vi "Append String to Error Source.vi"(4 "Append to Warning? (F)":bool, 6 "Prepend? (F)":bool, 8 "Error In":errorcluster, 9 "String to Append":string) -> (0 "Error Out":errorcluster)   [LabVIEW 2023]
doc: "Append or Prepend the specified message to the input error source string if error exists."
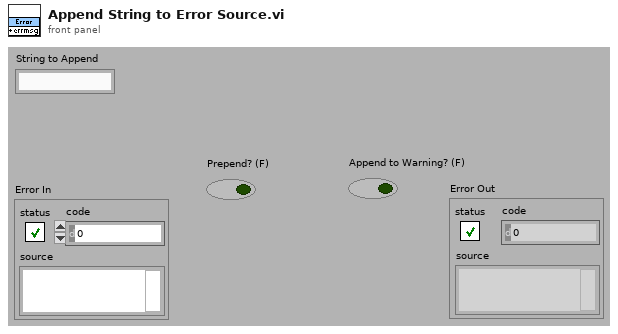
[diagram p1: front panel]
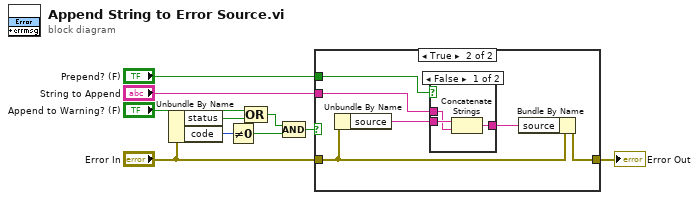
[diagram p0: block diagram]
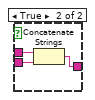
[diagram p3: hidden frame]
diagram:
  n1 = Unbundle By Name("Error In") -> ("status"=w10:bool, "code"=w7:i32)
  n2 = Not Equal To 0?(x=w7) -> (x != 0?=w6:bool)
  n3 = Compound Arithmetic op=OR("Append to Warning? (F)", w10) -> (w8:bool)
  n4 = Compound Arithmetic op=AND(w8, w6) -> (w5:bool)
  n5 = case shown="True" w5 {
    tunnel: "Error In" -> [w11 w17]
    tunnel: [w11 w16] -> w3
    tunnel: "Prepend? (F)" -> [_ w12]
    tunnel: "String to Append" -> [_ w13]
    frame False {
    }
    frame True {
      n6 = Unbundle By Name(w17) -> ("source"=w15:string)
      n7 = case shown="False" w12 {
        tunnel: w15 -> [w20 w23]
        tunnel: [w19 w21] -> w14
        tunnel: w13 -> [w18 w22]
        frame False {
          n8 = Concatenate Strings(w20, w18) -> (w19:string)
        }
        frame True {
          n9 = Concatenate Strings(w22, w23) -> (w21:string)
        }
      }
      n10 = Bundle By Name(cluster=w17, "source"=w14) -> (w16:errorcluster)
    }
  }
  "Error Out" <- w3
